vi "get_component_type_name.vi"(8 "error in (no error)":errorcluster, 11 "GeneralAnalyser in":refnum<class "GenericAnalyser.lvclass">) -> (0 "error out":errorcluster, 2 "component type":string, 3 "GeneralAnalyser out":refnum<class "GenericAnalyser.lvclass">)   [LabVIEW 2010, in "GenericAnalyser.lvclass"]
uses:
  GenericAnalyser.lvclass
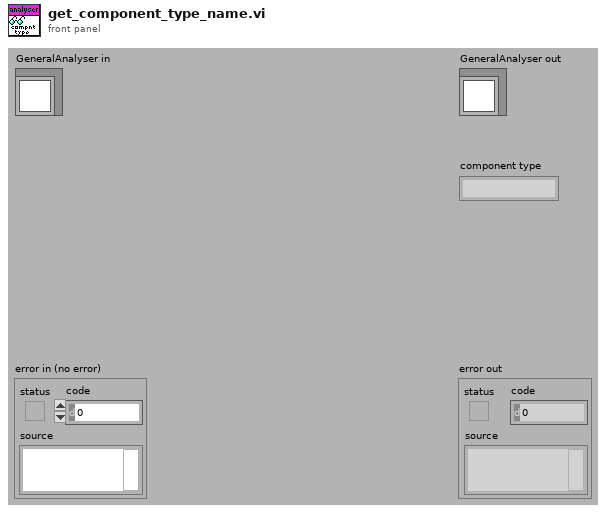
[diagram p1: front panel]
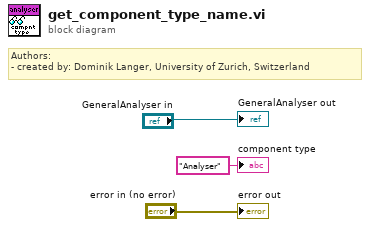
[diagram p0: block diagram]
diagram:
  # "Authors: \n- created by: Dominik Langer, University of Zurich, Switzerland"
  "error out" <- "error in (no error)"
  "GeneralAnalyser out" <- "GeneralAnalyser in"
  "component type" <- "Analyser" ("component type")
